vi "UDT_application_Get Data In.vi"() -> (3 "Unit Test Framework Results":T1)   [LabVIEW 2017]
doc: "Use this template to create a user-defined test VI. Define your test requirements and wire the results to the <b>Result (Test)</b> control. Do not modify the <b>Unit Test Framework Results</b> indicator."
uses:
  <vilib>/utf/common/utf_test_result_troll.ctl
  <vilib>/utf/common/utf_test_result.ctl
  <vilib>/utf/common/utf_test_result_failure.ctl
  <vilib>/utf/common/utf_test_comparison_operators.ctl
  <vilib>/utf/common/utf_vi_tag.ctl
  RT/TypeDefs/allData.ctl
  RT/TypeDefs/dataOut.ctl
  RT/TypeDefs/dataIn.ctl
  RT/SubVIs/FGVs/TypeDefs/DataFGVControl.ctl
  <vilib>/Control Software Solutions Ltd/UTF Helper/SubVIs/UTF Double Equals.vi
  <vilib>/Control Software Solutions Ltd/UTF Helper/SubVIs/UTF Boolean Equals.vi
  <vilib>/Control Software Solutions Ltd/UTF Helper/Unit Test Helper.lvlib
  <vilib>/utf/NI_UnitTestFramework.lvlib
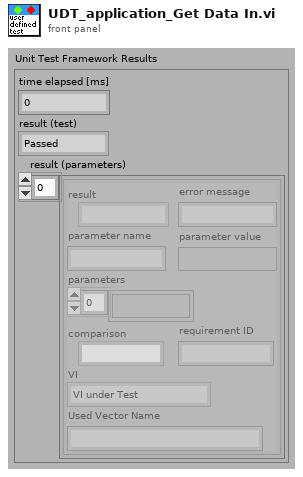
[diagram p1: front panel]
types:
  T1 = typedef "NI_UnitTestFramework.lvlib/utf_test_result_troll.ctl" = cluster{"time elapsed [ms]":u32, "result (test)":T2, "result (parameters)":T3[]}
  T2 = typedef "NI_UnitTestFramework.lvlib/utf_test_result.ctl" = enum16{"Passed", "Failed", "Error", "Skipped", "Not Processed"}
  T3 = typedef "NI_UnitTestFramework.lvlib/utf_test_result_failure.ctl" = cluster{"result":T2, "error message":string, "parameter name":string, "parameter value":variant, "parameters":variant[], "comparison":T4, "requirement ID":string, "VI":T5, "Used Vector Name":string}
  T4 = typedef "NI_UnitTestFramework.lvlib/utf_test_comparison_operators.ctl" = enum16{"=", "!=", ">", ">=", "<", "<=", "range", "symmetric tolerance", "asymmetric tolerance", "string contains", "string not contain", "array size", "string length", "array range", "by element", "array range (limit array)", "user-defined", "array contains", "array not contain", "vector length", "= (elm)", "!= (elm)", "= (case insensitive)", "!= (case insensitive)"}
  T5 = typedef "NI_UnitTestFramework.lvlib/utf_vi_tag.ctl" = enum16{"Setup VI", "VI under Test", "Teardown VI"}
  T6 = typedef "dataIn.ctl" = cluster{"Xtarget":dbl, "Ytarget":dbl, "Ztarget":dbl, "X_Attractor 1":dbl, "Y_Attractor 1":dbl, "Z_Attractor 1":dbl, "X_Attractor 2":dbl, "Y_Attractor 2":dbl, "Z_Attractor 2":dbl, "Traj Flag":bool, "DeadZone":dbl, "Assistance":bool, "Shutdown?":bool, "AssistanceLevel":dbl}
  T7 = typedef "DataFGVControl.ctl" = enum16{"Set Data", "Get Data"}
  T8 = typedef "allData.ctl" = cluster{"DataOut":T9, "DataIn":T6}
  T9 = typedef "dataOut.ctl" = cluster{"X0pos":dbl, "Y0pos":dbl, "Z0pos":dbl, "Fx":dbl, "Fy":dbl, "Fz":dbl, "Encoder1":i32, "Encoder2":i32, "Pot1":dbl, "Pot2":dbl, "Theta0":dbl, "Theta1":dbl, "X1pos":dbl, "Y1pos":dbl, "Z1pos":dbl, "X2pos":dbl, "Y2pos":dbl, "Z2pos":dbl, "ErrorOccurred":bool}
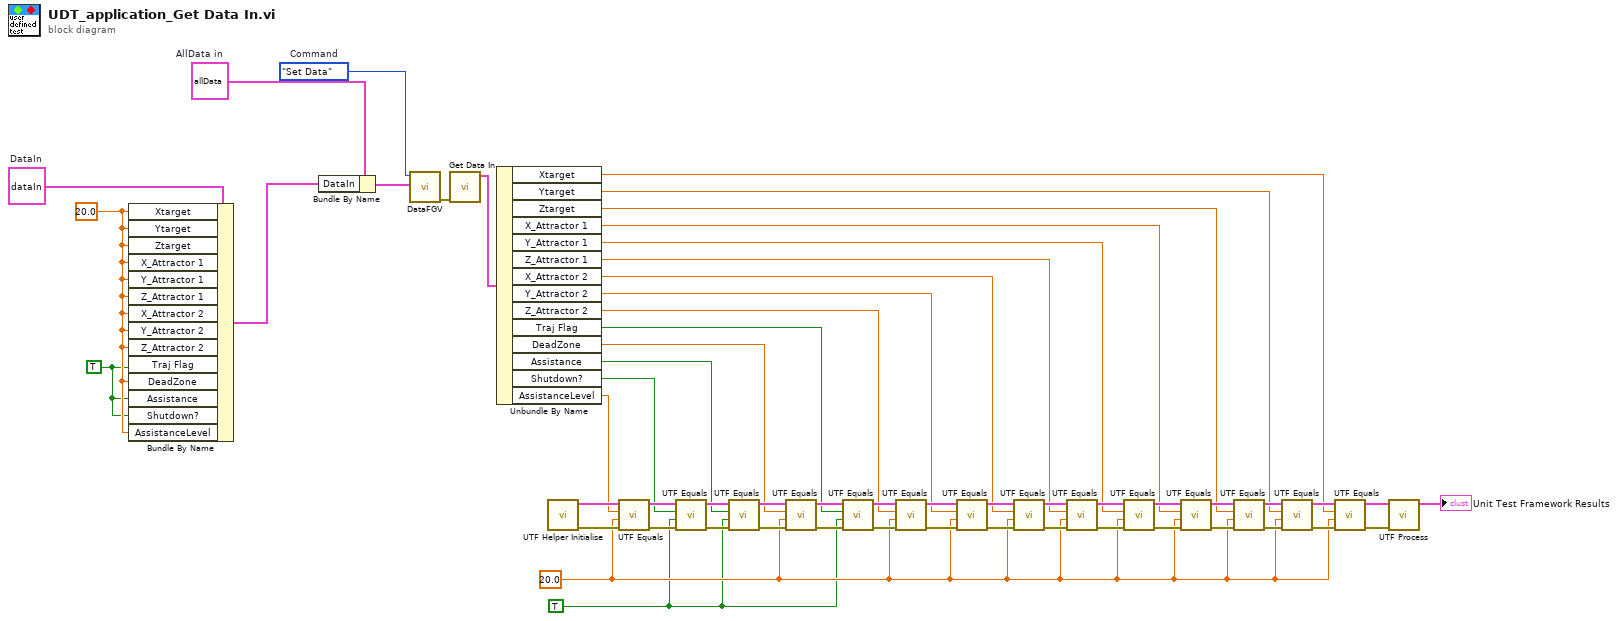
[diagram p0: block diagram]
diagram:
  w16 = TRUE ("Test Value")
  w17 = 20.0 ("Xtarget")
  w20 = T6 {"Xtarget"=0.0, "Ytarget"=0.0, "Ztarget"=0.0, "X_Attractor 1"=0.0, "Y_Attractor 1"=0.0, "Z_Attractor 1"=0.0, "X_Attractor 2"=0.0, "Y_Attractor 2"=0.0, "Z_Attractor 2"=0.0, "Traj Flag"=FALSE, "DeadZone"=0.0, "Assistance"=FALSE, "Shutdown?"=FALSE, "AssistanceLevel"=0.0}  # DataIn
  w22 = TRUE ("Test Value")
  w23 = 20.0 ("Xtarget")
  w56 = DataFGVControl."Set Data"  # Command
  w54 = T8 {"DataOut"={"X0pos"=0.0, "Y0pos"=0.0, "Z0pos"=0.0, "Fx"=0.0, "Fy"=0.0, "Fz"=0.0, "Encoder1"=0, "Encoder2"=0, "Pot1"=0.0, "Pot2"=0.0, "Theta0"=0.0, "Theta1"=0.0, "X1pos"=0.0, "Y1pos"=0.0, "Z1pos"=0.0, "X2pos"=0.0, "Y2pos"=0.0, "Z2pos"=0.0, "ErrorOccurred"=FALSE}, "DataIn"={"Xtarget"=0.0, "Ytarget"=0.0, "Ztarget"=0.0, "X_Attractor 1"=0.0, "Y_Attractor 1"=0.0, "Z_Attractor 1"=0.0, "X_Attractor 2"=0.0, "Y_Attractor 2"=0.0, "Z_Attractor 2"=0.0, "Traj Flag"=FALSE, "DeadZone"=0.0, "Assistance"=FALSE, "Shutdown?"=FALSE, "AssistanceLevel"=0.0}}  # AllData in
  n1 = Bundle By Name(cluster=w20, "Xtarget"=w17, "Ytarget"=w17, "Ztarget"=w17, "X_Attractor 1"=w17, "Y_Attractor 1"=w17, "Z_Attractor 1"=w17, "X_Attractor 2"=w17, "Y_Attractor 2"=w17, "Z_Attractor 2"=w17, "Traj Flag"=w16, "DeadZone"=w17, "Assistance"=w16, "Shutdown?"=w16, "AssistanceLevel"=w17) -> (w19:T6)
  n2 = Bundle By Name(cluster=w54, "DataIn"=w19) -> (w18:T8)
  n3 = call "DataFGV.vi"("AllData in"=w18, "Command"=w56) -> ("error out"=w55:errorcluster)  [unwired: 8 in, 1 out]
  n4 = call "Get Data In.vi"("error in (no error)"=w55) -> ("DataIn"=w15:T6)  [unwired: 9 in, 1 out]
  n5 = Unbundle By Name(w15) -> ("Xtarget"=w1:dbl, "Ytarget"=w2:dbl, "Ztarget"=w3:dbl, "X_Attractor 1"=w4:dbl, "Y_Attractor 1"=w5:dbl, "Z_Attractor 1"=w6:dbl, "X_Attractor 2"=w7:dbl, "Y_Attractor 2"=w8:dbl, "Z_Attractor 2"=w9:dbl, "Traj Flag"=w10:bool, "DeadZone"=w11:dbl, "Assistance"=w12:bool, "Shutdown?"=w13:bool, "AssistanceLevel"=w14:dbl)
  n6 = call <vilib>:"UTF Helper Initialise.vi"() -> ("error out"=w50:errorcluster, "results array"=w51:T3[])  [unwired: 10 in]
  n7 = call-poly <vilib>:"UTF Equals.vi"("error in (no error)"=w50, "Test Value"=w23, "Input"=w14, "Input Results"=w51) -> ("error out"=w49:errorcluster, "Output Results"=w52:T3[])  [unwired: 6 in]
  n8 = call-poly <vilib>:"UTF Equals.vi"("error in (no error)"=w49, "Test Value"=w22, "Input"=w13, "Input Results"=w52) -> ("error out"=w48:errorcluster, "Output Results"=w53:T3[])  [unwired: 6 in]
  n9 = call-poly <vilib>:"UTF Equals.vi"("error in (no error)"=w48, "Test Value"=w22, "Input"=w12, "Input Results"=w53) -> ("error out"=w47:errorcluster, "Output Results"=w46:T3[])  [unwired: 6 in]
  n10 = call-poly <vilib>:"UTF Equals.vi"("error in (no error)"=w47, "Test Value"=w23, "Input"=w11, "Input Results"=w46) -> ("error out"=w42:errorcluster, "Output Results"=w45:T3[])  [unwired: 6 in]
  n11 = call-poly <vilib>:"UTF Equals.vi"("error in (no error)"=w42, "Test Value"=w22, "Input"=w10, "Input Results"=w45) -> ("error out"=w43:errorcluster, "Output Results"=w44:T3[])  [unwired: 6 in]
  n12 = call-poly <vilib>:"UTF Equals.vi"("error in (no error)"=w43, "Test Value"=w23, "Input"=w9, "Input Results"=w44) -> ("error out"=w41:errorcluster, "Output Results"=w40:T3[])  [unwired: 6 in]
  n13 = call-poly <vilib>:"UTF Equals.vi"("error in (no error)"=w41, "Test Value"=w23, "Input"=w8, "Input Results"=w40) -> ("error out"=w39:errorcluster, "Output Results"=w30:T3[])  [unwired: 6 in]
  n14 = call-poly <vilib>:"UTF Equals.vi"("error in (no error)"=w39, "Test Value"=w23, "Input"=w7, "Input Results"=w30) -> ("error out"=w38:errorcluster, "Output Results"=w31:T3[])  [unwired: 6 in]
  n15 = call-poly <vilib>:"UTF Equals.vi"("error in (no error)"=w38, "Test Value"=w23, "Input"=w6, "Input Results"=w31) -> ("error out"=w37:errorcluster, "Output Results"=w32:T3[])  [unwired: 6 in]
  n16 = call-poly <vilib>:"UTF Equals.vi"("error in (no error)"=w37, "Test Value"=w23, "Input"=w5, "Input Results"=w32) -> ("error out"=w36:errorcluster, "Output Results"=w33:T3[])  [unwired: 6 in]
  n17 = call-poly <vilib>:"UTF Equals.vi"("error in (no error)"=w36, "Test Value"=w23, "Input"=w4, "Input Results"=w33) -> ("error out"=w35:errorcluster, "Output Results"=w34:T3[])  [unwired: 6 in]
  n18 = call-poly <vilib>:"UTF Equals.vi"("error in (no error)"=w35, "Test Value"=w23, "Input"=w3, "Input Results"=w34) -> ("error out"=w29:errorcluster, "Output Results"=w28:T3[])  [unwired: 6 in]
  n19 = call-poly <vilib>:"UTF Equals.vi"("error in (no error)"=w29, "Test Value"=w23, "Input"=w2, "Input Results"=w28) -> ("error out"=w26:errorcluster, "Output Results"=w27:T3[])  [unwired: 6 in]
  n20 = call-poly <vilib>:"UTF Equals.vi"("error in (no error)"=w26, "Test Value"=w23, "Input"=w1, "Input Results"=w27) -> ("error out"=w24:errorcluster, "Output Results"=w25:T3[])  [unwired: 6 in]
  n21 = call <vilib>:"UTF Process.vi"("error in (no error)"=w24, "results array"=w25) -> ("Unit Test Framework Results"=→"Unit Test Framework Results":T1)  [unwired: 9 in]
